vi "Read Pulse Recorder Configuration.vi"(8 "error in (no error)":errorcluster, 11 "RP I-V in":refnum<class "RP I-V.lvclass">) -> (0 "error out":errorcluster, 2 "Configuration":T1={"Pre-trigger duration"=0.01, "Post-trigger duration"=0.1, "Rate"=1000000.0, "Ranges"=[10.0], "Re-name channels"=[], "Active channels"="0:1", "External clock"=FALSE} {"Rate" format="%#_8pHz"; "Post-trigger duration" format="%#_6ps"; "Pre-trigger duration" format="%#_6ps"; "Ranges" format="%#_6pV"}, 3 "RP I-V out":refnum<class "RP I-V.lvclass">)   [LabVIEW 2016, in "RP I-V.lvclass"]
uses:
  RP I-V.lvclass
  D:/github/Measure_core/Template Module/Template Module.lvclass
  NHMFL_Core/Libraries/Instruments/Pulse Driver/Pusle Driver Configuration.ctl
  Measure_core/Template Module/Template Module.lvclass/Template Module.ctl
  NHMFL_Core/Libraries/Red Pitaya/RP Core/Rep Pitaya I-V driver/RP I-V Configuration.ctl
  NHMFL_Core/Libraries/Red Pitaya/Waform generation/I-V parameters.ctl
  Measure_core/Template Module/Read Configuration.vi
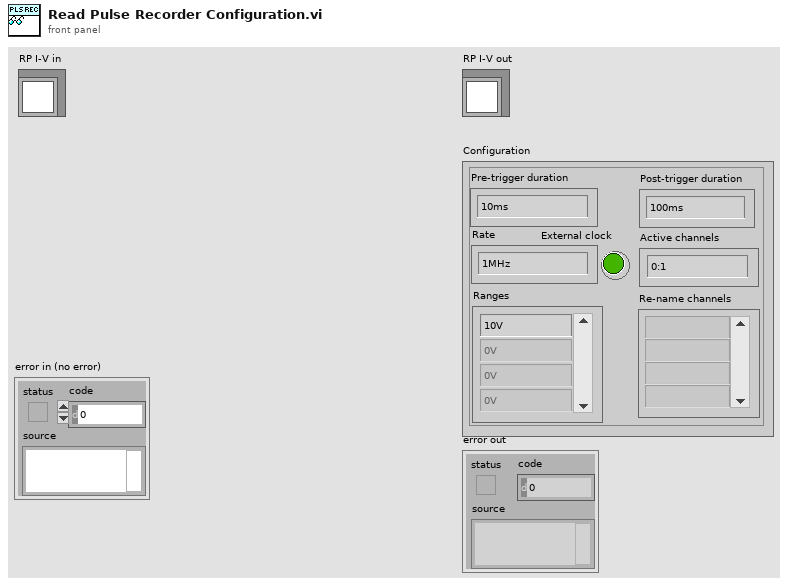
[diagram p1: front panel]
types:
  T1 = typedef "Pusle Driver Configuration.ctl" = cluster{"Pre-trigger duration":dbl, "Post-trigger duration":dbl, "Rate":dbl, "Ranges":dbl[], "Re-name channels":string[], "Active channels":string, "External clock":bool}
  T2 = typedef "RP I-V Configuration.ctl" = cluster{"Recorder":T1, "I-V parameters":T3}
  T3 = typedef "I-V parameters.ctl" = cluster{"Start magnitude":dbl, "Magnitude increment":dbl, "Number of pulses":i32, "Baseline length":dbl, "Ramp length":dbl, "Top  length":dbl, "Threshold ":dbl}
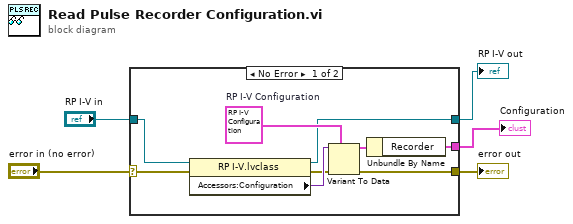
[diagram p0: block diagram]
diagram:
  n1 = case shown="No Error" "error in (no error)" {
    selector: "error in (no error)" -> [w9 w15]
    tunnel: [w8 w15] -> w3
    tunnel: [w7 w16] -> w1
    tunnel: "RP I-V in" -> [w12 w16]
    tunnel: [w6 _] -> w2
    frame No Error {
      w11 = T2 {"Recorder"={"Pre-trigger duration"=0.0, "Post-trigger duration"=0.0, "Rate"=0.0, "Ranges"=[], "Re-name channels"=[], "Active channels"="", "External clock"=FALSE}, "I-V parameters"={"Start magnitude"=0.0, "Magnitude increment"=0.0, "Number of pulses"=0, "Baseline length"=0.0, "Ramp length"=0.0, "Top  length"=0.0, "Threshold "=0.0}}  # RP I-V Configuration
      n2 = property class="RP I-V.lvclass"(reference=w12, error in=w9) -> (reference out=w7:refnum<class "RP I-V.lvclass">, error out=w13:errorcluster, "Accessors:Configuration"=w14:variant)
      n3 = Variant To Data(error in=w13, type=w11, Variant=w14) -> (data=w10:T2, error out=w8:errorcluster)
      n4 = Unbundle By Name(w10) -> ("Recorder"=w6:T1)
    }
    frame Error {
    }
  }
  "error out" <- w3
  "RP I-V out" <- w1
  "Configuration" <- w2
